vi "Sonar.vi"(8 "error in (no error)":errorcluster) -> (0 "error out":errorcluster, 3 "CM":fxp<+,64,16>)   [LabVIEW 2018]
panel:
  in  "stop":bool
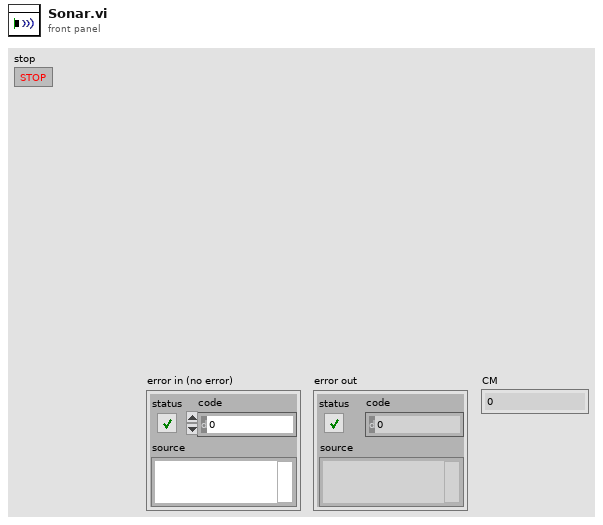
[diagram p1: front panel]
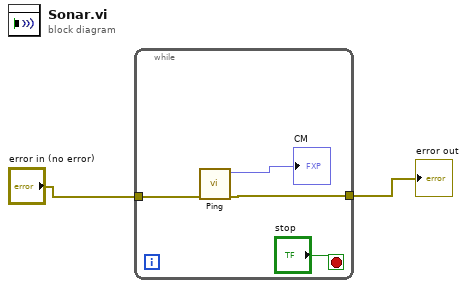
[diagram p0: block diagram]
diagram:
  n1 = while {
    tunnel: "error in (no error)" -> [w5]
    tunnel: [w4] -> w1
    stop <- "stop" stop-if-true
    n2 = call <vilib>:"Ping.vi"("error in (no error)"=w5) -> ("error out"=w4:errorcluster, "CM"=→"CM":fxp<+,64,16>)  [unwired: 8 in, 1 out]
  }
  "error out" <- w1
